vi "FPVdll.vi"(8 "error in (no error)":errorcluster, 11 "Inputs":cluster{"t":dbl, "D":dbl, "p":dbl, "z":dbl[]}) -> (0 "error out":errorcluster, 3 "f":dbl)   [LabVIEW 2015]
doc: "subroutine FPV (t,D,p,z,f)\n\nCompute the supercompressibility factor, Fpv.\n\nINPUTS:\nt -- temperature [K]\nD -- molar density [mol/L]\np -- pressure [kPa]\nz -- composition [array of mol frac]\n\nOUTPUTS:\nf -- Fpv = sqrt[Z(60 F, 14.73 psia)/Z(T,P)]"
uses:
  REFPROP.dll
panel:
  # "REFPROP-FPVdll.vi"
  # "void  FPVdll(double *t, double *D, double *p, double *z, double *f)"
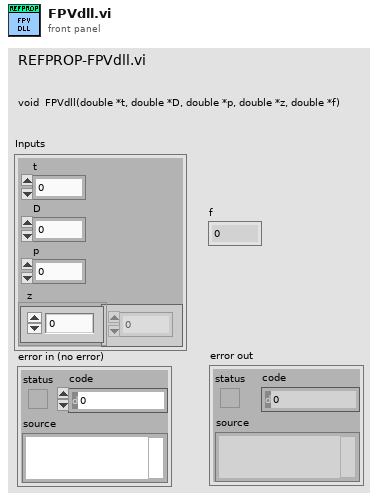
[diagram p1: front panel]
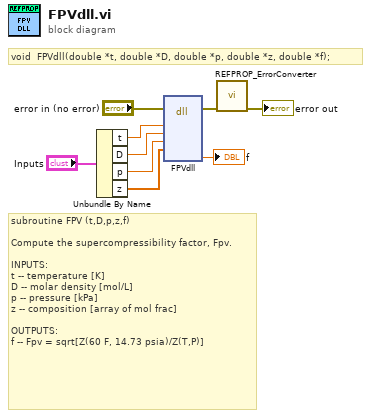
[diagram p0: block diagram]
diagram:
  # "void  FPVdll(double *t, double *D, double *p, double *z, double *f);"
  # "subroutine FPV (t,D,p,z,f)\n\nCompute the supercompressibility factor, Fpv.\n\nINPUTS:\nt -- temperature [K]\nD -- molar density [mol/L]\np -- pressure [kPa]\nz -- composition [array of mol frac]\n\nOUTPUTS:\nf -- Fpv = sqrt[Z(60 F, 14.73 psia)/Z(T,P)]"
  n1 = Unbundle By Name("Inputs") -> ("t"=w4:dbl, "D"=w3:dbl, "p"=w2:dbl, "z"=w1:dbl[])
  n2 = dll-call lib="C:/Users/lauria/Desktop/REFPROP 10 LabVIEW Wrapper BETA/REFPROP/REFPROP.*" fn="FPVdll"(error in="error in (no error)", "t"=w4, "D"=w3, "p"=w2, "z"=w1) -> (error out=w8:errorcluster, "f"=→"f":dbl)  [unwired: 8 in, 1 out]
  n3 = call "REFPROP_ErrorConverter.vi"("error in (no error)"=w8) -> ("error out"=→"error out":errorcluster)  [unwired: 10 in]
